vi "Configure List.vi"(6 "List Points (0)":dbl[](array[numeric]), 7 "List Count (1)":i32=1, 8 "error in (no error)":errorcluster, 9 "List Type (0:Dwell Time)":u16(ring) items=["Dwell Time", "Frequency", "Frequency Slew Rate", "Phase", "TTL Trigger", "Voltage", "Voltage Slew Rate"], 10 "Enable Auto List Sequencing (T: Enable)":bool=TRUE, 11 "VISA resource name":refnum<visa-resource-name>) -> (0 "error out":errorcluster, 3 "VISA resource name out":refnum<visa-resource-name>)   [LabVIEW 2010, in "California Instruments iX Series.lvlib"]
doc: "Configures the list sequences of output changes with rapid, precise timing and synchronized with internal and external signals."
uses:
  <instrlib>/California Instruments iX Series/California Instruments iX Series.lvlib
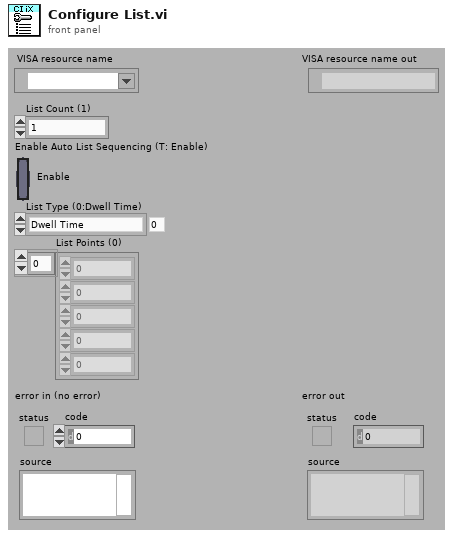
[diagram p1: front panel]
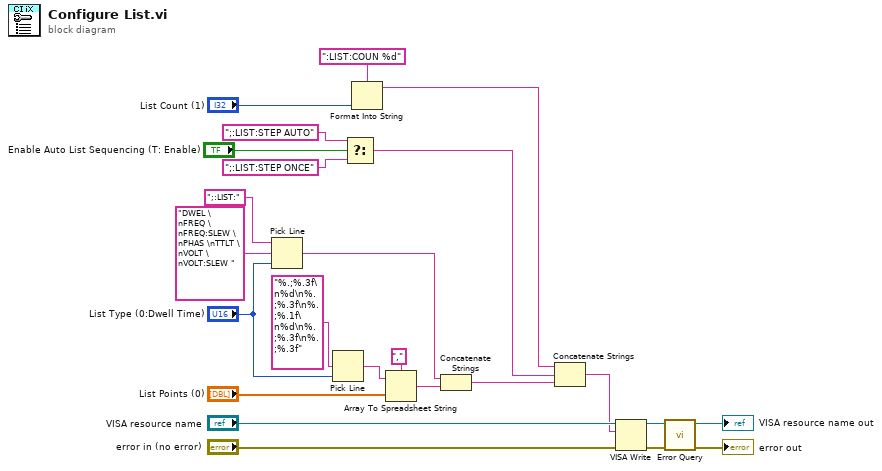
[diagram p0: block diagram]
diagram:
  n1 = Pick Line(string ("")=";:LIST:", multi-line string="DWEL \nFREQ \nFREQ:SLEW \nPHAS \nTTLT \nVOLT \nVOLT:SLEW ", line index="List Type (0:Dwell Time)") -> (output string=w9:string)
  n2 = Pick Line(multi-line string="%.;%.3f\n%d\n%.;%.3f\n%.;%.1f\n%d\n%.;%.3f\n%.;%.3f" ("f"), line index="List Type (0:Dwell Time)") -> (output string=w1:string)  [unwired: 1 in]
  n3 = Select(t=";:LIST:STEP AUTO", s="Enable Auto List Sequencing (T: Enable)", f=";:LIST:STEP ONCE") -> (s? t:f=w6:string)
  n4 = Format Into String(format string=":LIST:COUN %d", "List Count (1)") -> (resulting string=w7:string)  [unwired: 2 in, 1 out]
  n5 = Array To Spreadsheet String(delimiter (Tab)=",", array="List Points (0)", 3:w1) -> (spreadsheet string=w8:string)
  n6 = Concatenate Strings(w9, w8) -> (w5:string)
  n7 = Concatenate Strings(w7, w6, w5) -> (w4:string)
  n8 = VISA Write(VISA resource name="VISA resource name", write buffer=w4, error in (no error)="error in (no error)") -> (VISA resource name out=w22:refnum<visa-resource-name>, error out=w21:errorcluster)  [unwired: 1 out]
  n9 = call <instrlib>:"Error Query.vi"("error in (no error)"=w21, "VISA resource name"=w22) -> ("error out"=→"error out":errorcluster, "VISA resource name out"=→"VISA resource name out":refnum<visa-resource-name>)  [unwired: 6 in, 2 out]
